vi "Day-1.vi"() -> ()   [LabVIEW 2017]
panel:
  out "Numeric 2":dbl
  in  "Numeric 4":dbl
  out "Numeric 3":dbl
  out "output":dbl
  in  "Numeric":dbl
  # "(Day-1)"
  # "Basic's of LabVIEW"
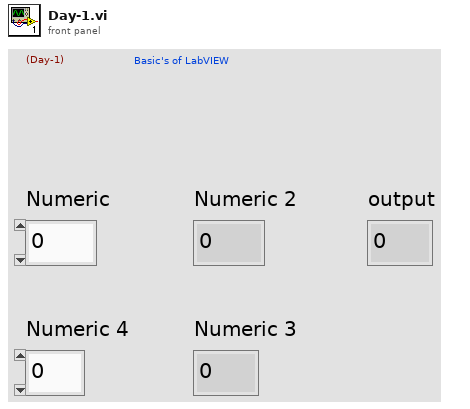
[diagram p1: front panel]
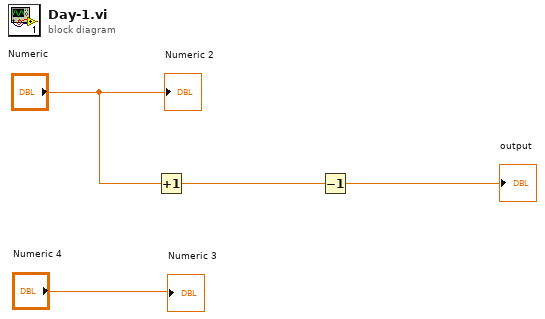
[diagram p0: block diagram]
diagram:
  n1 = Increment(x="Numeric") -> (x+1=w4:dbl)
  n2 = Decrement(x=w4) -> (x-1=→"output":dbl)
  "Numeric 3" <- "Numeric 4"
  "Numeric 2" <- "Numeric"
